vi "Andor Ixon_Cam.vi"(4 "Frames in sequence":u32, 6 "Image in":variant, 7 "Camera-specific in":variant, 8 "Save path":path, 9 "Capture mode":enum16{"Single frame", "Sequence"}(ring), 10 "Exposure time (s)":dbl, 11 "Operation":T2(ring)) -> (3 "Status":T1, 5 "Camera-specific out":variant)   [LabVIEW 2012]
uses:
  <userlib>/atmcd64d.llb/Shutter_type typedef.ctl
  <vilib>/vision/Image Controls.llb/IMAQ Image.ctl
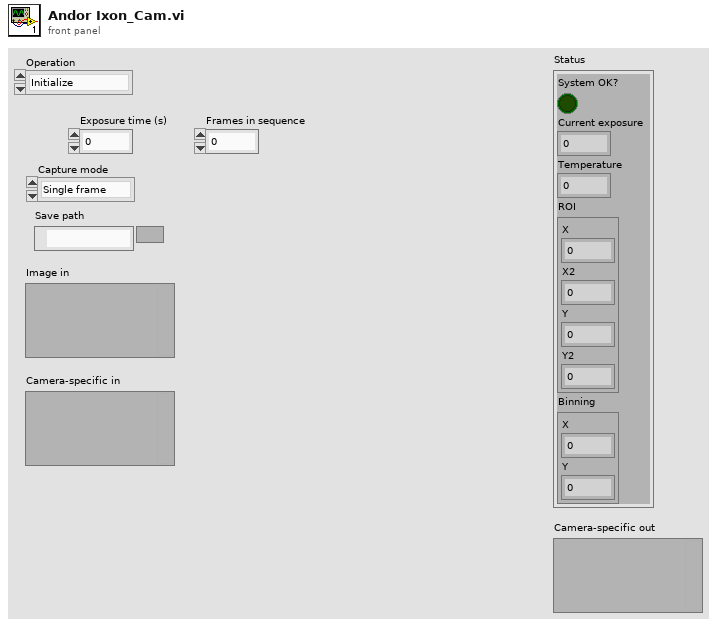
[diagram p1: front panel]
types:
  T1 = cluster{"System OK?":bool, "Current exposure":dbl, "Temperature":dbl, "ROI":cluster{"X":u32, "X2":u32, "Y":u32, "Y2":u32}, "Binning":cluster{"X":u32, "Y":u32}}
  T2 = enum16{"Initialize", "Shut down", "Set capture mode", "Set exposure", "Trigger and read", "Get status", "Other settings"}
  T3 = typedef "IMAQ Image.ctl" = refnum<image>
  T4 = cluster{"New Image":T3, "Image":refnum<vi>, "FPS target":dbl}
  T5 = enum16{"open", "replace", "create", "open or create", "replace or create", "replace or create with confirmation"}
  T6 = typedef "Shutter_type typedef.ctl" = enum16{"TTL Low", "TTL High"}
  T7 = typedef "Error Code Enum typedef.ctl" = enum32{"N/A (0)", "DRV_ERROR_CODES", "DRV_SUCCESS", "DRV_VXDNOTINSTALLED", "DRV_ERROR_SCAN", "DRV_ERROR_CHECK_SUM", "DRV_ERROR_FILELOAD", "DRV_UNKNOWN_FUNC", "DRV_ERROR_VXD_INIT", "DRV_ERROR_ADDRESS", "DRV_ERROR_PAGELOCK", "DRV_ERROR_PAGEUNLOCK", "DRV_ERROR_BOARDTEST", "DRV_ERROR_ACK", "DRV_ERROR_UP_FIFO", "DRV_ERROR_PATTERN", "N/A (16)", "DRV_ACQUISITION_ERRORS", "DRV_ACQ_BUFFER", "DRV_ACQ_DOWNFIFO_FULL", "DRV_PROC_UNKONWN_INSTRUCTION", "DRV_ILLEGAL_OP_CODE", "DRV_KINETIC_TIME_NOT_MET", "DRV_ACCUM_TIME_NOT_MET", "DRV_NO_NEW_DATA", "N/A (25)", "DRV_SPOOLERROR", "N/A (27)", "N/A (28)", "N/A (29)", "N/A (30)", "N/A (31)", "N/A (32)", "DRV_TEMPERATURE_CODES", "DRV_TEMPERATURE_OFF", "DRV_TEMPERATURE_NOT_STABILIZED", "DRV_TEMPERATURE_STABILIZED", "DRV_TEMPERATURE_NOT_REACHED", "DRV_TEMPERATURE_OUT_RANGE", "DRV_TEMPERATURE_NOT_SUPPORTED", "DRV_TEMPERATURE_DRIFT", "N/A (41)", "N/A (42)", "N/A (43)", "N/A (44)", "N/A (45)", "N/A (46)", "N/A (47)", "N/A (48)", "DRV_GENERAL_ERRORS", "DRV_INVALID_AUX", "DRV_COF_NOTLOADED", "DRV_FPGAPROG", "DRV_FLEXERROR", "DRV_GPIBERROR", "N/A (55)", "N/A (56)", "N/A (57)", "N/A (58)", "N/A (59)", "N/A (60)", "N/A (61)", "N/A (62)", "N/A (63)", "DRV_DATATYPE", "DRV_DRIVER_ERRORS", "DRV_P1INVALID", "DRV_P2INVALID", "DRV_P3INVALID", "DRV_P4INVALID", "DRV_INIERROR", "DRV_COFERROR", "DRV_ACQUIRING", "DRV_IDLE", "DRV_TEMPCYCLE", "DRV_NOT_INITIALIZED", "DRV_P5INVALID", "DRV_P6INVALID", "DRV_INVALID_MODE", "DRV_INVALID_FILTER", "DRV_I2CERRORS", "DRV_I2CDEVNOTFOUND", "DRV_I2CTIMEOUT", "DRV_P7INVALID", "N/A (84)", "N/A (85)", "N/A (86)", "N/A (87)", "N/A (88)", "N/A (89)", "DRV_IOCERROR", "DRV_VRMVERSIONERROR"}
  T8 = cluster{"File refnum":refnum<file>, "Image File Directory":cluster{cluster{"Field":u16, "Type":u16, "Count":u32, "Value / Offset":u32, "Add IFD Offset?":bool}[], cluster{"Data":u32[], "Add offset?":bool}[]}, "Big endian?":bool, "IFD Offset Size":u32}
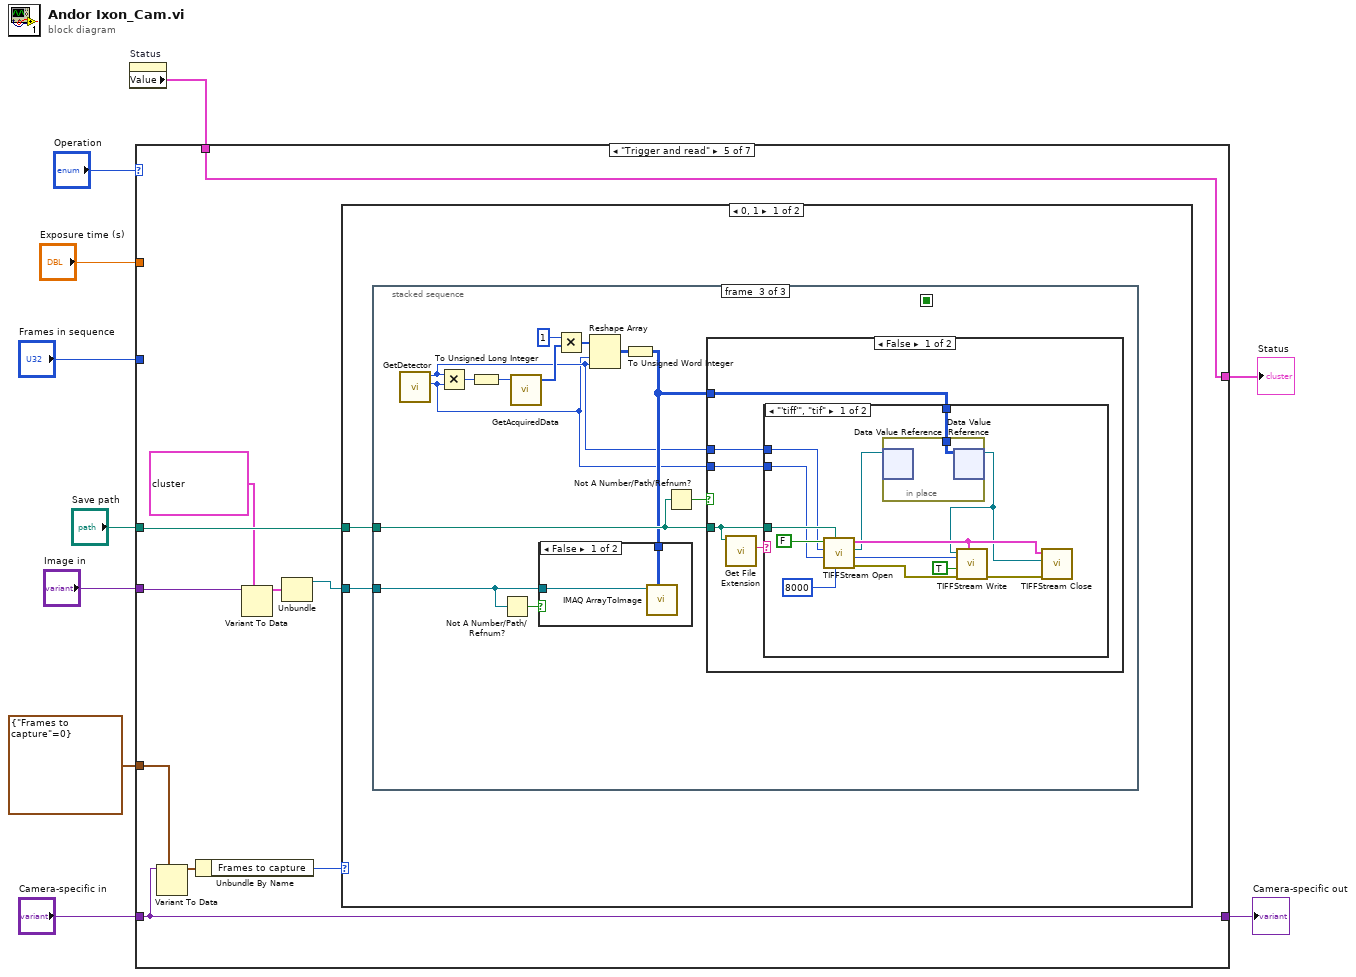
[diagram p0: block diagram]
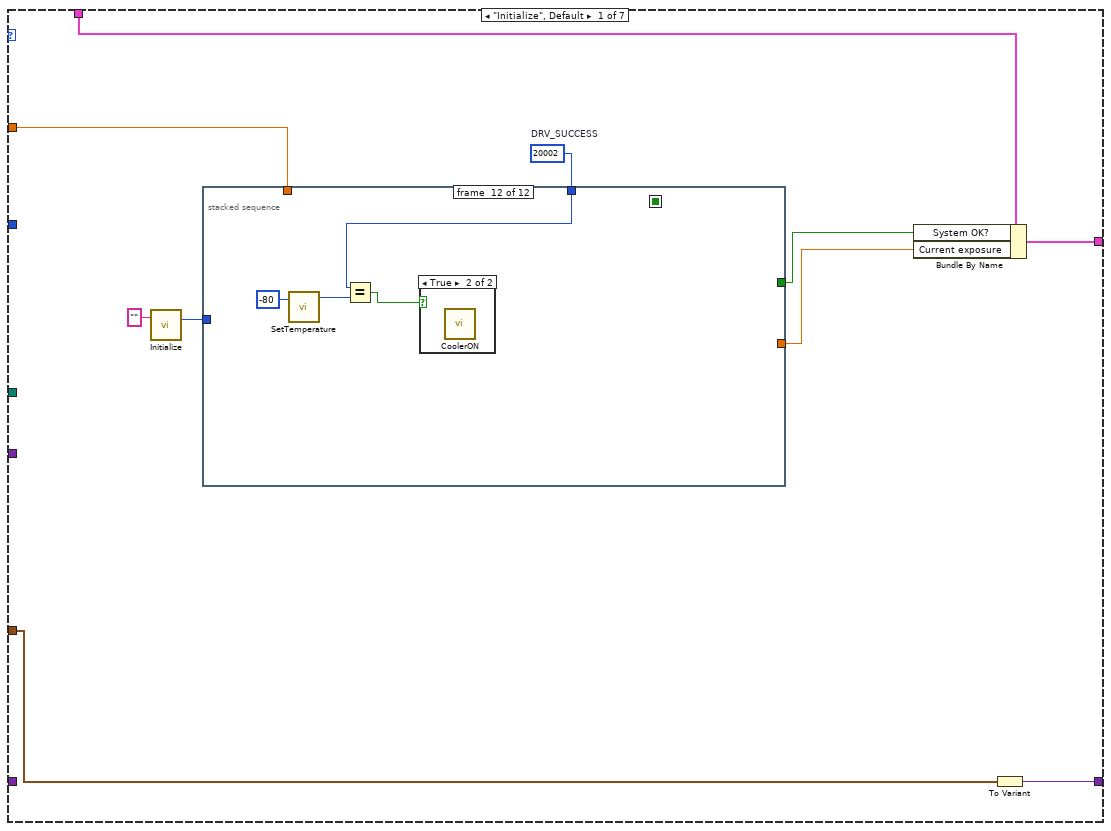
[diagram p2: hidden frame]
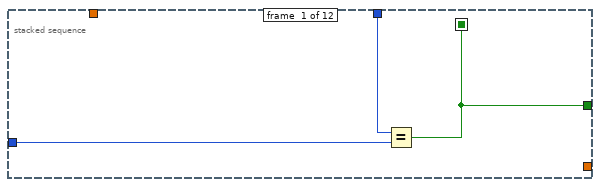
[diagram p3: hidden frame]
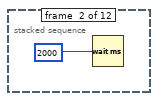
[diagram p4: hidden frame]
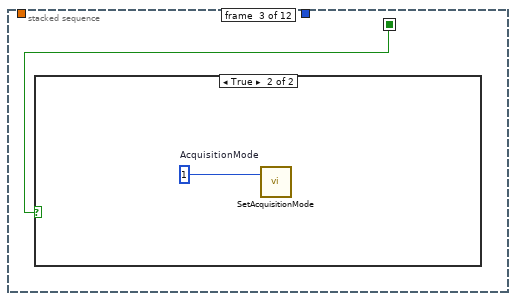
[diagram p5: hidden frame]
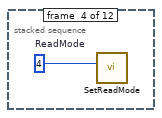
[diagram p7: hidden frame]
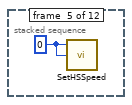
[diagram p8: hidden frame]
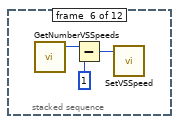
[diagram p9: hidden frame]
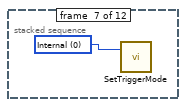
[diagram p10: hidden frame]
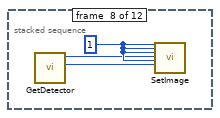
[diagram p11: hidden frame]
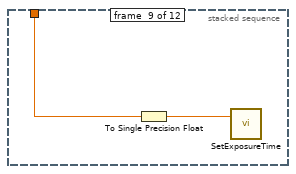
[diagram p12: hidden frame]
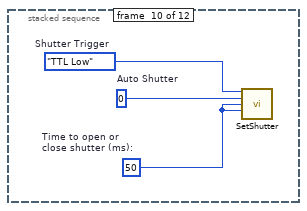
[diagram p13: hidden frame]
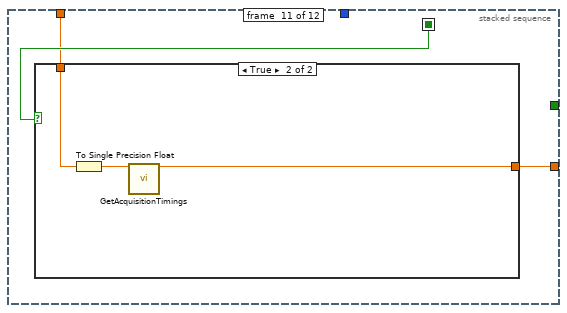
[diagram p14: hidden frame]
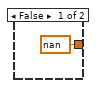
[diagram p15: hidden frame]
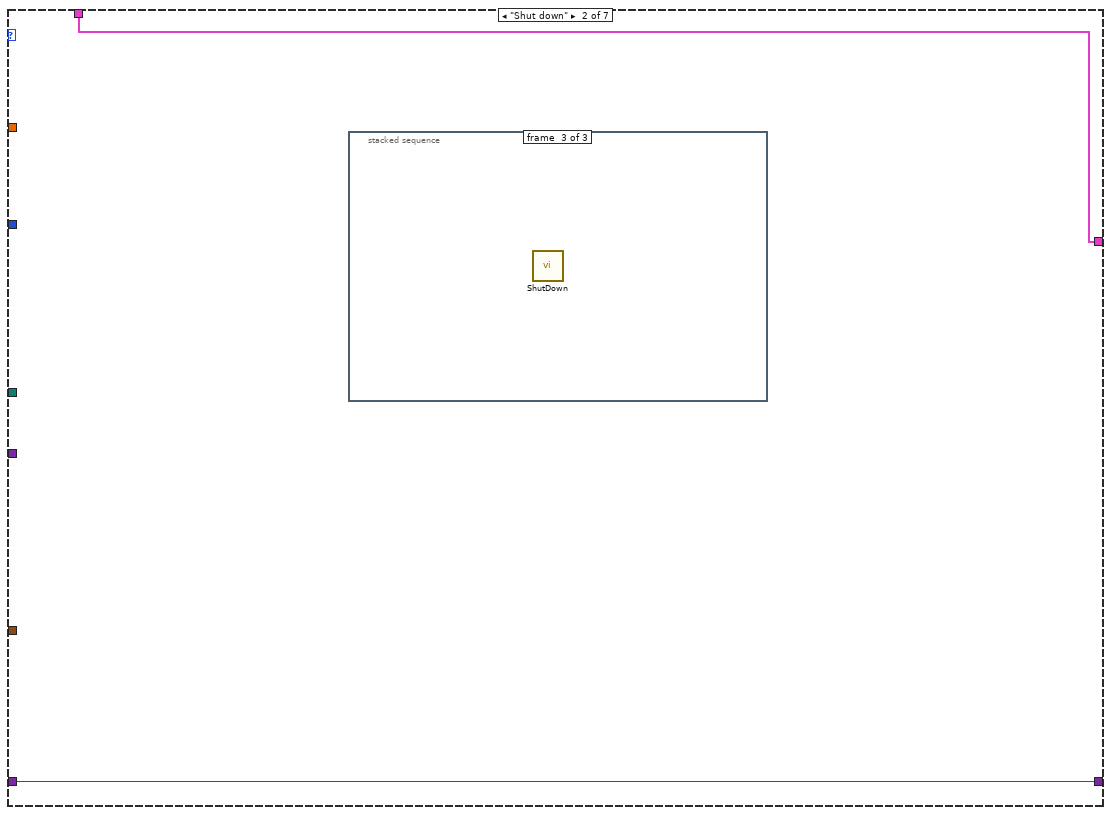
[diagram p17: hidden frame]
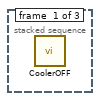
[diagram p18: hidden frame]
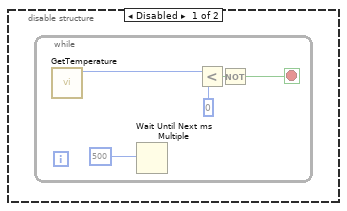
[diagram p20: hidden frame]
diagram:
  n1 = property on="Status" class="Clust (strict)"() -> ("Value"=w8:T1)  [unwired: 2 in, 2 out]
  n2 = case shown="\"Trigger and read\"" "Operation" {
    tunnel: "Exposure time (s)" -> [w17 _ _ w77 _ _ _]
    tunnel: w8 -> [w16 w53 w67 w79 w92 w149 w151]
    tunnel: [w15 w53 w67 w76 w92 w148 w151] -> w7
    tunnel: "Save path" -> [_ _ _ _ w91 _ _]
    tunnel: "Image in" -> [_ _ _ _ w84 _ _]
    tunnel: [w11 w52 w62 w74 w90 w143 w150] -> w4
    tunnel: "Camera-specific in" -> [_ w52 w65 w74 w90 w143 w150]
    tunnel: cluster{"Frames to capture":u32} {"Frames to capture"=0} -> [w12 _ w64 _ w89 _ _]
    tunnel: "Frames in sequence" -> [_ _ w59 _ _ _ _]
    frame "Initialize", Default {
      w18 = 20002  # DRV_SUCCESS
      n3 = call <userlib>:"Initialize.vi"("directory (\"\")"="" ("directory (\"\")")) -> ("DLL error code"=w19:u32)  [unwired: 1 in, 1 out]
      n4 = stacked-sequence {
        seq-local: [w21 _ _ _ _ _ _ _ _ _ _ _] -> [_ _ w25 _ _ _ _ _ _ _ w43 _]
        tunnel: w17 -> [_ _ _ _ _ _ _ _ w37 _ w42 _]
        tunnel: w18 -> [w23 _ _ _ _ _ _ _ _ _ _ w49]
        tunnel: w19 -> [w22 _ _ _ _ _ _ _ _ _ _ _]
        tunnel: [w21 _ _ _ _ _ _ _ _ _ _ _] -> w14
        tunnel: [_ _ _ _ _ _ _ _ _ _ w41 _] -> w13
        frame #0 {
          n5 = Equal?(x=w23, y=w22) -> (x = y?=w21:bool)
        }
        frame #1 {
          n6 = Wait (ms)(milliseconds to wait=u32 2000) -> ()  [unwired: 1 out]
        }
        frame #2 {
          n7 = case shown="True" w25 {
            frame False {
            }
            frame True {
              w26 = u16 1  # AcquisitionMode
              n8 = call <userlib>:"SetAcquisitionMode.vi"("mode"=w26) -> ()  [unwired: 1 in, 2 out]
            }
          }
        }
        frame #3 {
          w27 = u16 4  # ReadMode
          n9 = call <userlib>:"SetReadMode.vi"("mode"=w27) -> ()  [unwired: 1 in, 2 out]
        }
        frame #4 {
          w28 = 0
          n10 = call <userlib>:"SetHSSpeed.vi"("index"=w28, "type"=w28) -> ()  [unwired: 2 in, 2 out]
        }
        frame #5 {
          n11 = call <userlib>:"GetNumberVSSpeeds.vi"() -> ("number"=w31:i32)  [unwired: 3 in, 2 out]
          n12 = Subtract(x=w31, y=1) -> (x-y=w29:i32)
          n13 = call <userlib>:"SetVSSpeed.vi"("index"=w29) -> ()  [unwired: 1 in, 2 out]
        }
        frame #6 {
          w32 = u32 0 items=["Internal", "External"] ("Trigger")
          n14 = call <userlib>:"SetTriggerMode.vi"("mode"=w32) -> ()  [unwired: 1 in, 2 out]
        }
        frame #7 {
          w35 = 1 ("hbin")
          n15 = call <userlib>:"GetDetector.vi"() -> ("ypixels"=w33:i32, "xpixels"=w34:i32)  [unwired: 4 in, 2 out]
          n16 = call <userlib>:"SetImage.vi"("hbin"=w35, "vbin"=w35, "hstart"=w35, "hend"=w34, "vstart"=w35, "vend"=w33) -> ()  [unwired: 20 in, 2 out]
        }
        frame #8 {
          n17 = To Single Precision Float(number=w37) -> (single precision float=w36:sgl)
          n18 = call <userlib>:"SetExposureTime.vi"("time"=w36) -> ()  [unwired: 1 in, 2 out]
        }
        frame #9 {
          w40 = 50  # Time to open or close shutter (ms):
          w38 = Shutter_type_typedef."TTL Low"  # Shutter Trigger
          w39 = 0  # Auto Shutter
          n19 = call <userlib>:"SetShutter.vi"("type"=w38, "mode"=w39, "closingtime"=w40, "openingtime"=w40) -> ()  [unwired: 10 in, 2 out]
        }
        frame #10 {
          n20 = case shown="True" w43 {
            tunnel: w42 -> [_ w47]
            tunnel: [sgl nan ("exposure") w46] -> w41
            frame False {
            }
            frame True {
              n21 = To Single Precision Float(number=w47) -> (single precision float=w45:sgl)
              n22 = call <userlib>:"GetAcquisitionTimings.vi"("exposure input"=w45) -> ("exposure"=w46:sgl)  [unwired: 10 in, 4 out]
            }
          }
        }
        frame #11 {
          n23 = call <userlib>:"SetTemperature.vi"("temperature"=-80) -> ("DLL error code"=w50:u32)  [unwired: 1 in, 1 out]
          n24 = Equal?(x=w49, y=w50) -> (x = y?=w48:bool)
          n25 = case shown="True" w48 {
            frame False {
            }
            frame True {
              n26 = call <userlib>:"CoolerON.vi"() -> ()  [unwired: 2 in, 2 out]
            }
          }
        }
      }
      n27 = Bundle By Name(cluster=w16, "System OK?"=w14, "Current exposure"=w13) -> (w15:T1)
      n28 = To Variant(anything=w12) -> (Variant=w11:variant)
    }
    frame "Shut down" {
      n29 = stacked-sequence {
        frame #0 {
          n30 = call <userlib>:"CoolerOFF.vi"() -> ()  [unwired: 2 in, 2 out]
        }
        frame #1 {
          # "Wait for temperature to get above freezing"
          n31 = disable-structure shown="Enabled" {
            frame Disabled {
              n32 = while {
                stop <- w54 stop-if-true
                n33 = call <userlib>:"GetTemperature.vi"() -> ("temperature"=w55:i32)  [unwired: 4 in, 3 out]
                n34 = Wait Until Next ms Multiple(millisecond multiple=u32 500) -> ()  [unwired: 1 out]
                n35 = Less?(x=w55, y=i16 0) -> (x < y?=w57:bool)
                n36 = Not(x=w57) -> (.not. x?=w54:bool)
              }
            }
            frame Enabled {
            }
          }
        }
        frame #2 {
          n37 = call <userlib>:"ShutDown.vi"() -> ()  [unwired: 2 in, 2 out]
        }
      }
    }
    frame "Set capture mode" {
      n38 = Variant To Data(type=w64, Variant=w65) -> (data=w63:cluster{"Frames to capture":u32})  [unwired: 1 in, 1 out]
      n39 = case shown="\"Single frame\", Default" "Capture mode" {
        tunnel: [u32 0 ("Frames in sequence") w70] -> w60
        tunnel: w59 -> [_ w70]
        frame "Single frame", Default {
          w69 = u16 1  # AcquisitionMode
          n40 = call <userlib>:"SetAcquisitionMode.vi"("mode"=w69) -> ()  [unwired: 1 in, 2 out]
        }
        frame "Sequence" {
          w73 = u16 3  # AcquisitionMode
          n41 = call <userlib>:"SetAcquisitionMode.vi"("mode"=w73) -> ("error out"=w72:errorcluster)  [unwired: 1 in, 1 out]
          n42 = call <userlib>:"SetFrameTransferMode.vi"("error in (no error)"=w72, "mode"=enum16{"OFF", "ON"}."ON") -> ()  [unwired: 2 out]
        }
      }
      n43 = Bundle By Name(cluster=w63, "Frames to capture"=w60) -> (w61:cluster{"Frames to capture":u32})
      n44 = To Variant(anything=w61) -> (Variant=w62:variant)
    }
    frame "Set exposure" {
      n45 = To Single Precision Float(number=w77) -> (single precision float=w78:sgl)
      n46 = stacked-sequence {
        tunnel: w78 -> [w80 w82]
        tunnel: [_ w81] -> w75
        frame #0 {
          n47 = call <userlib>:"SetExposureTime.vi"("time"=w80) -> ()  [unwired: 1 in, 2 out]
        }
        frame #1 {
          n48 = call <userlib>:"GetAcquisitionTimings.vi"("exposure input"=w82) -> ("exposure"=w81:sgl)  [unwired: 10 in, 4 out]
        }
      }
      n49 = Bundle By Name(cluster=w79, "Current exposure"=w75) -> (w76:T1)
    }
    frame "Trigger and read" {
      n50 = Variant To Data(type=w89, Variant=w90) -> (data=w88:cluster{"Frames to capture":u32})  [unwired: 1 in, 1 out]
      n51 = Unbundle By Name(w88) -> ("Frames to capture"=w87:u32)
      n52 = Variant To Data(type=T4 {"New Image"=refnum, "Image"=refnum, "FPS target"=0.0} ("output cluster"), Variant=w84) -> (data=w86:T4)  [unwired: 1 in, 1 out]
      n53 = Unbundle(w86) -> ("New Image"=w83:T3)  [unwired: 2 out]
      n54 = case shown="0, 1" w87 {
        tunnel: w91 -> [w94 _]
        tunnel: w83 -> [w93 _]
        frame 0, 1 {
          n55 = stacked-sequence {
            seq-local: [w97 _ _] -> [_ w98 _]
            tunnel: w94 -> [_ _ w109]
            tunnel: w93 -> [_ _ w107]
            frame #0 {
              w95 = 20002  # DRV_SUCCESS
              n56 = call <userlib>:"StartAcquisition.vi"() -> ("DLL error code"=w96:u32)  [unwired: 2 in, 1 out]
              n57 = Equal?(x=w95, y=w96) -> (x = y?=w97:bool)
            }
            frame #1 {
              n58 = case shown="True" w98 {
                frame False {
                }
                frame True {
                  n59 = while {
                    stop <- w101 continue-if-true
                    w100 = u16 72  # DRV ACQUIRING
                    n60 = call <userlib>:"GetStatus.vi"() -> ("status"=w99:T7)  [unwired: 3 in, 2 out]
                    n61 = Wait Until Next ms Multiple(millisecond multiple=u32 25) -> ()  [unwired: 1 out]
                    n62 = Equal?(x=w99, y=w100) -> (x = y?=w101:bool)
                  }
                }
              }
            }
            frame #2 {
              n63 = call <userlib>:"GetDetector.vi"() -> ("ypixels"=w103:i32, "xpixels"=w104:i32)  [unwired: 4 in, 2 out]
              n64 = Multiply(x=w104, y=w103) -> (x*y=w115:i32)
              n65 = To Unsigned Long Integer(number=w115) -> (unsigned 32bit integer=w111:u32)
              n66 = Not A Number/Path/Refnum?(number/path/refnum=w107) -> (NaN/Path/Refnum?=w106:bool)
              n67 = call <userlib>:"GetAcquiredData.vi"("size"=w111) -> ("array"=w113:i32[])  [unwired: 2 in, 2 out]
              n68 = Multiply(x=1, y=w113) -> (x*y=w112:i32[])
              n69 = Reshape Array(w112, w103, w104) -> (w108:i32[][])
              n70 = To Unsigned Word Integer(number=w108) -> (unsigned 16bit integer=w105:u16[][])
              n71 = case shown="False" w106 {
                tunnel: w107 -> [w117 _]
                tunnel: w105 -> [w116 _]
                frame False {
                  n72 = call "IMAQ ArrayToImage"("Image Pixels (U16)"=w116, "Image"=w117) -> ()  [unwired: 8 in, 2 out]
                }
                frame True {
                }
              }
              n73 = Not A Number/Path/Refnum?(number/path/refnum=w109) -> (NaN/Path/Refnum?=w110:bool)
              n74 = case shown="False" w110 {
                tunnel: w109 -> [w121 _]
                tunnel: w105 -> [w122 _]
                tunnel: w104 -> [w119 _]
                tunnel: w103 -> [w118 _]
                frame False {
                  n75 = call <vilib>:"Get File Extension.vi"("file"=w121) -> ("lowercase file extension"=w120:string)  [unwired: 7 in, 3 out]
                  n76 = case shown="\"'tiff'\", \"tif\"" w120 {
                    tunnel: w121 -> [w135 w142]
                    tunnel: w122 -> [w125 w140]
                    tunnel: w119 -> [w133 _]
                    tunnel: w118 -> [w132 _]
                    frame "'tiff'", "tif" {
                      n77 = call "TIFFStream Open.vi"("Bytes per strip"=u32 8000, "File path"=w135, "Height Pixels"=w132, "Width Pixels"=w133, "Big endian?"=FALSE) -> ("error out"=w129:errorcluster, "Next IFD Offset"=w127:u32, "Image data reference"=w126:refnum<data-value>, "File data"=w131:T8)  [unwired: 3 in]
                      n78 = in-place {
                        in-place-border: w125 -> [w136]
                        n79 = in-place-dvr #1(w126) -> ()  [unwired: 2 out]
                        n80 = in-place-dvr #1(w136) -> (w124:refnum<data-value>)  [unwired: 1 out]
                      }
                      n81 = call "TIFFStream Write.vi"("File data"=w131, "error in (no error)"=w129, "Last image in file?"=TRUE, "IFD Offset"=w127, "Image data reference"=w124) -> ("error out"=w130:errorcluster)  [unwired: 5 in, 1 out]
                      n82 = call "TIFFStream Close.vi"("error in (no error)"=w130, "Image data reference"=w124, "File data"=w131) -> ()  [unwired: 8 in, 1 out]
                    }
                    frame "dat", Default {
                      n83 = Open/Create/Replace File(file path (use dialog)=w142, operation (0:open)=T5."replace or create") -> (refnum out=w141:refnum<file>)  [unwired: 4 in, 2 out]
                      n84 = Write to Binary File(file (use dialog)=w141, data=w140, 5:FALSE ("prepend array or string size? (T)")) -> (refnum out=w138:refnum<file>)  [unwired: 3 in, 2 out]
                      n85 = Close File(refnum=w138) -> ()  [unwired: 1 in, 2 out]
                    }
                  }
                }
                frame True {
                }
              }
            }
          }
        }
        frame 2, Default {
        }
      }
    }
    frame "Get status" {
      w145 = 20002  # DRV_SUCCESS
      n86 = call <userlib>:"GetTemperature.vi"() -> ("status"=w146:T7, "temperature"=w147:i32)  [unwired: 4 in, 2 out]
      n87 = Equal?(x=w145, y=w146) -> (x = y?=w144:bool)
      n88 = Bundle By Name(cluster=w149, "System OK?"=w144, "Temperature"=w147) -> (w148:T1)
    }
    frame "Other settings" {
      n89 = call "Andor Ixon_Settings.vi"() -> ()  [unwired: 12 in]
    }
  }
  "Status" <- w7
  "Camera-specific out" <- w4
